vi "GetPersonnel.vi"(7 "Room Commands":T1, 8 "error in (no error)":errorcluster, 11 "PUID":string) -> (0 "error out":errorcluster, 2 "JSON":string)   [LabVIEW 2015, in "PersonnelRestApi.lvlib"]
uses:
  PersonnelRestApi.lvlib
  TypeDef/GetPersonnelCommands.ctl
  TypeDef/FGVAction.ctl
  <vilib>/httpClient/LabVIEWHTTPClient.lvlib
  RoomRestApi.lvlib
panel:
  out "URL":string
  out "headers":string
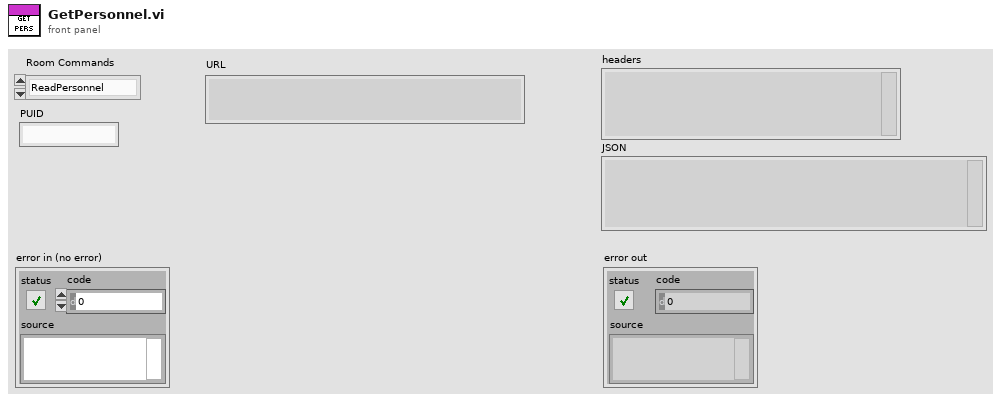
[diagram p1: front panel]
types:
  T1 = typedef "PersonnelRestApi.lvlib/GetPersonnelCommands.ctl" = enum16{"ReadPersonnel", "ReadName", "ReadRole", "ReadRequests", "ReadPUIDs", "ReadAllPersonnel"}
  T2 = typedef "RoomRestApi.lvlib/FGVAction.ctl" = enum16{"Get", "Set"}
  T3 = typedef "LabVIEWHTTPClient.lvlib/ClientHandle.ctl" = refnum<k1>
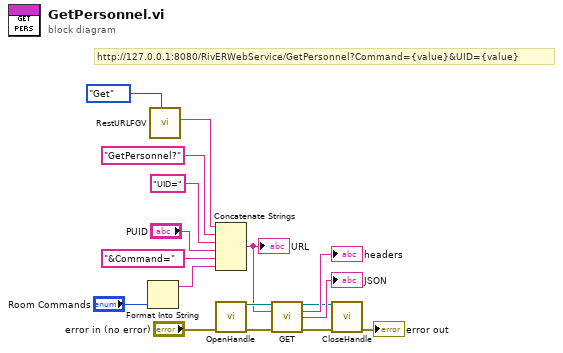
[diagram p0: block diagram]
diagram:
  # "http://127.0.0.1:8080/RivERWebService/GetPersonnel?Command={value}&UID={value}"
  n1 = Format Into String("Room Commands") -> (resulting string=w2:string)  [unwired: 3 in, 1 out]
  n2 = call "RestURLFGV.vi"("Action"=FGVAction."Get") -> ("URL"=w6:string)  [unwired: 9 in, 1 out]
  n3 = Concatenate Strings(w6, "GetPersonnel?" ("string"), "UID=" ("string"), "PUID", "&Command=" ("string"), w2) -> (w7:string)
  "URL" <- w7
  n4 = call <vilib>:"OpenHandle.vi"("error in (no error)"="error in (no error)") -> ("client handle out"=w17:T3, "error out"=w12:errorcluster)  [unwired: 13 in]
  n5 = call <vilib>:"GET.vi"("client handle"=w17, "url"=w7, "error in (no error)"=w12) -> ("client handle out"=w14:T3, "headers"=→"headers":string, "body"=→"JSON":string, "error out"=w13:errorcluster)  [unwired: 9 in]
  n6 = call <vilib>:"CloseHandle.vi"("client handle"=w14, "error in (no error)"=w13) -> ("error out"=→"error out":errorcluster)  [unwired: 13 in]
